vi "Transistor curves gate sweep.vi"() -> ()   [LabVIEW 2014]
uses:
  Environmental Chamber LabVIEW and Instruments/Drivers and Software/LabVIEW 8.2 Drivers/keithley_24xx/Keithley 24XX/Public/Data/Read (Single Point).vi
  <vilib>/Utility/file.llb/Write To Spreadsheet File (string).vi
  Environmental Chamber LabVIEW and Instruments/Drivers and Software/keithley_24xx/Keithley 24XX/Keithley 24XX.lvlib
  Environmental Chamber LabVIEW and Instruments/Drivers and Software/keithley_6430/Keithley 6430/Keithley 6430.lvlib
panel:
  out "new file path":path
  in  "Stop Button":bool
  in  "Measure settings":T1={"source low (V)"=0.0, "source high (V)"=0.3, "source points"=30.0, "gate low (V)"=0.0, "gate high (V)"=0.3, "gate points"=30.0} {"gate low (V)" min=-190.0 max=190.0}
  out "2420 IV curve":cluster{"X":dbl[], "Y":dbl[]}[](graph)
  # "6430 = bias\n2420 = source-drain"
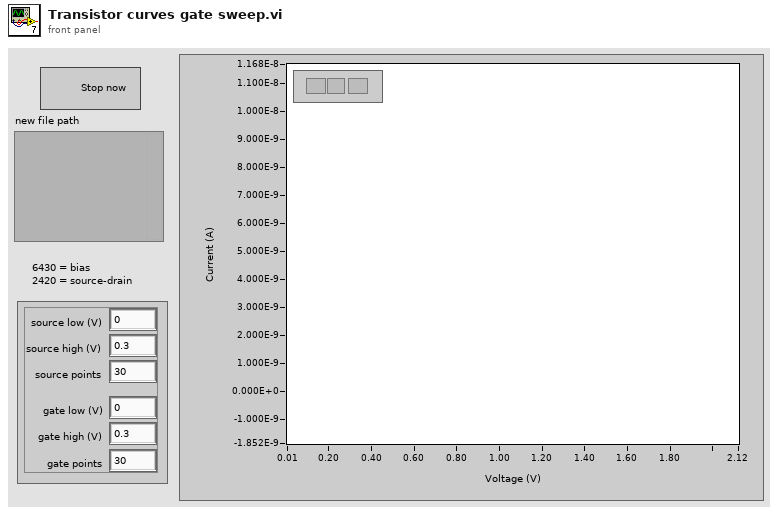
[diagram p1: front panel]
types:
  T1 = cluster{"source low (V)":dbl, "source high (V)":dbl, "source points":dbl, "gate low (V)":dbl, "gate high (V)":dbl, "gate points":dbl}
  T2 = enum16{"open", "open or create", "create or replace", "create", "open (read only)"}
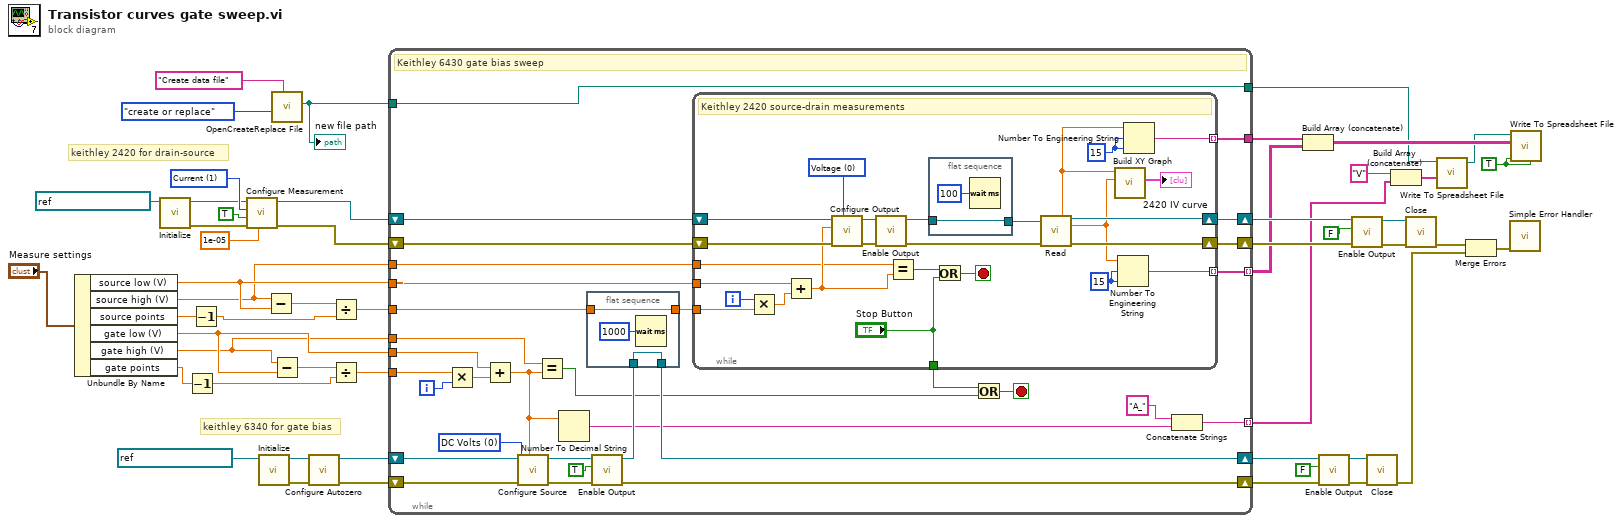
[diagram p0: block diagram]
diagram:
  w22 = TRUE ("transpose? (no:F)")
  w43 = u16 1 items=["Volts", "Current", "Resistance"] ("Function (0: Volts)")
  # "keithley 6340 for gate bias"
  # "keithley 2420 for drain-source"
  n1 = Unbundle By Name("Measure settings") -> ("source low (V)"=w13:dbl, "source high (V)"=w12:dbl, "source points"=w6:dbl, "gate low (V)"=w11:dbl, "gate high (V)"=w10:dbl, "gate points"=w4:dbl)
  n2 = call "Initialize.vi"("VISA resource name"=refnum<visa-resource-name> "GPIB1::24::INSTR") -> ("error out"=w39:errorcluster, "VISA resource name out"=w40:refnum<visa-resource-name>)  [unwired: 9 in]
  n3 = Decrement(x=w4) -> (x-1=w3:dbl)
  n4 = Decrement(x=w6) -> (x-1=w5:dbl)
  n5 = call "Configure Measurement.vi"("Manual Range (1.0)"=1e-05, "error in (no error)"=w39, "Enable Auto Range (T:Enable)"=TRUE, "Function (0: Volts)"=w43, "VISA resource name"=w40) -> ("error out"=w42:errorcluster, "VISA resource name out"=w41:refnum<visa-resource-name>)  [unwired: 5 in]
  n6 = call "Initialize.vi"("VISA resource name"=refnum<visa-resource-name> "GPIB2::19::INSTR") -> ("error out"=w34:errorcluster, "VISA resource name out"=w35:refnum<visa-resource-name>)  [unwired: 4 in, 5 out]
  n7 = Subtract(x=w12, y=w13) -> (x-y=w51:dbl)
  n8 = call "OpenCreateReplace File.vi"("prompt"="Create data file", "function (open:0)"=T2."create or replace") -> ("new file path"=w1:path)  [unwired: 6 in, 3 out]
  "new file path" <- w1
  n9 = Subtract(x=w10, y=w11) -> (x-y=w23:dbl)
  n10 = call "Configure Autozero.vi"("error in (no error)"=w34, "VISA resource name"=w35) -> ("error out"=w24:errorcluster, "VISA resource name out"=w25:refnum<visa-resource-name>)  [unwired: 8 in]
  n11 = Divide(x=w51, y=w5) -> (x/y=w50:dbl)
  n12 = Divide(x=w23, y=w3) -> (x/y=w19:dbl)
  n13 = while {
    tunnel: w12 -> [w83]
    tunnel: w13 -> [w82]
    tunnel: w50 -> [w61]
    tunnel: [w54] -> w2 mode=indexing
    tunnel: [w71] -> w21
    shift-right: [w80] -> w45
    shift-left: w42 -> [w79]
    shift-right: [w62] -> w30
    shift-left: w25 -> [w76]
    shift-right: [w64] -> w29
    shift-left: w24 -> [w75]
    shift-right: [w81] -> w46
    shift-left: w41 -> [w72]
    tunnel: w19 -> [w69]
    tunnel: w11 -> [w68]
    tunnel: w10 -> [w65]
    tunnel: [w59] -> w15 mode=indexing
    tunnel: [w52] -> w9
    tunnel: w1 -> [w52]
    i -> [w70]
    stop <- w57 stop-if-true
    w78 = u16 0 items=["DC Volts", "DC Current"] ("Source Function (0: DC Volts)")
    # "Keithley 6430 gate bias sweep"
    n14 = Multiply(x=w69, y=w70) -> (x*y=w67:dbl)
    n15 = Add(x=w68, y=w67) -> (x+y=w66:dbl)
    n16 = call "Configure Source.vi"("V-Source Level [V]"=w66, "error in (no error)"=w75, "Source Function (0: DC Volts)"=w78, "VISA resource name"=w76) -> ("error out"=w73:errorcluster, "VISA resource name out"=w74:refnum<visa-resource-name>)  [unwired: 6 in]
    n17 = Equal?(x=w65, y=w66) -> (x = y?=w58:bool)
    n18 = Number To Decimal String(number=w66) -> (decimal integer string=w55:string)  [unwired: 1 in]
    n19 = flat-sequence {
      tunnel: w63 -> [w85]
      tunnel: [w85] -> w62
      tunnel: w61 -> [w84]
      tunnel: [w84] -> w60
      frame #0 {
        n20 = Wait (ms)(milliseconds to wait=u32 1000 ("value")) -> ()  [unwired: 1 out]
      }
    }
    n21 = call "Enable Output.vi"("error in (no error)"=w73, "Enable Output (F:Off)"=TRUE ("Output (F:Off)"), "VISA resource name"=w74) -> ("error out"=w64:errorcluster, "VISA resource name out"=w63:refnum<visa-resource-name>)  [unwired: 7 out]
    n22 = while {
      tunnel: [w105] -> w59 mode=indexing
      shift-right: [w111] -> w80
      shift-left: w79 -> [w110]
      shift-right: [w112] -> w81
      shift-left: w72 -> [w109]
      tunnel: w60 -> [w91]
      tunnel: w82 -> [w102]
      tunnel: [w101] -> w71 mode=indexing
      tunnel: w83 -> [w93]
      tunnel: ["Stop Button"] -> w56
      i -> [w92]
      stop <- w89 stop-if-true
      w98 = i16 15 ("precision (6)")
      w99 = i16 15 ("precision (6)")
      w106 = u16 0 items=["Voltage", "Current"] ("Source Mode  (0: Voltage)")
      # "Keithley 2420 source-drain measurements"
      n23 = Multiply(x=w92, y=w91) -> (x*y=w100:dbl)
      n24 = Add(x=w102, y=w100) -> (x+y=w94:dbl)
      n25 = call "Configure Output.vi"("Source Mode  (0: Voltage)"=w106, "error in (no error)"=w110, "Output Level (0)"=w94, "VISA resource name"=w109) -> ("error out"=w108:errorcluster, "VISA resource name out"=w107:refnum<visa-resource-name>)  [unwired: 6 in]
      n26 = call "Enable Output.vi"("error in (no error)"=w108, "VISA resource name"=w107) -> ("error out"=w90:errorcluster, "VISA resource name out"=w104:refnum<visa-resource-name>)  [unwired: 8 in]
      n27 = Equal?(x=w93, y=w94) -> (x = y?=w88:bool)
      n28 = flat-sequence {
        tunnel: [w114] -> w103
        tunnel: w104 -> [w114]
        frame #0 {
          n29 = Wait (ms)(milliseconds to wait=u32 100) -> ()  [unwired: 1 out]
        }
      }
      n30 = Or(x=w88, y="Stop Button") -> (x .or. y?=w89:bool)
      n31 = call-poly "Read.vi"("VISA resource name"=w103, "error in (no error)"=w90) -> ("Voltage"=w96:sgl, "VISA resource name out"=w112:refnum<visa-resource-name>, "Current"=w97:sgl, "error out"=w111:errorcluster)  [unwired: 7 in, 3 out]
      n32 = call "Build XY Graph"("Y Input"=w97, "X Input"=w96) -> ("XY Graph"=→"2420 IV curve":cluster{"X":dbl[], "Y":dbl[]}[])  [unwired: 8 in, 1 out]
      n33 = Number To Engineering String(2:w99, 3:w99, 4:w97) -> (0:w105:string)  [unwired: 1 in]
      n34 = Number To Engineering String(2:w98, 3:w98, 4:w96) -> (0:w101:string)  [unwired: 1 in]
    }
    n35 = Or(x=w56, y=w58) -> (x .or. y?=w57:bool)
    n36 = Concatenate Strings("A_" ("string"), w55) -> (w54:string)
  }
  n37 = Build Array (concatenate)(w21, w15) -> (w20:string[][])
  n38 = call "Enable Output.vi"("error in (no error)"=w29, "Enable Output (F:Off)"=FALSE ("Output (F:Off)"), "VISA resource name"=w30) -> ("error out"=w31:errorcluster, "VISA resource name out"=w32:refnum<visa-resource-name>)  [unwired: 7 out]
  n39 = call "Enable Output.vi"("error in (no error)"=w45, "Enable Output (T: Enable)"=FALSE, "VISA resource name"=w46) -> ("error out"=w47:errorcluster, "VISA resource name out"=w49:refnum<visa-resource-name>)  [unwired: 7 in]
  n40 = call "Close.vi"("error in (no error)"=w31, "VISA resource name"=w32) -> ("error out"=w27:errorcluster)  [unwired: 9 out]
  n41 = Build Array (concatenate)("V", w2) -> (w17:string[])
  n42 = call "Close.vi"("error in (no error)"=w47, "VISA resource name"=w49) -> ("error out"=w28:errorcluster)  [unwired: 9 in]
  n43 = call-poly <vilib>:"Write To Spreadsheet File.vi"("1D data"=w17, "file path (dialog if empty)"=w9) -> ("new file path (Not A Path if cancelled)"=w16:path)  [unwired: 6 in]
  n44 = Merge Errors(w28, w27) -> (w26:errorcluster)
  n45 = call <vilib>:"Simple Error Handler.vi"("error in (no error)"=w26) -> ()  [unwired: 4 in, 5 out]
  n46 = call-poly <vilib>:"Write To Spreadsheet File.vi"("transpose? (no:F)"=w22, "append to file? (new file:F)"=w22, "2D data"=w20, "file path (dialog if empty)"=w16) -> ()  [unwired: 4 in, 1 out]
